vi "Send Command.vi"(8 "error in (no error)":errorcluster, 10 "write buffer":string, 11 "VISA resource name In":refnum<visa-resource-name>) -> (0 "error out":errorcluster, 3 "VISA resource name out":refnum<visa-resource-name>)   [LabVIEW 2017, in "Newport 1830-C.lvlib"]
doc: "Sends a command using the VISA drivers then waits sepecified ms."
uses:
  Newport 1830-C.lvlib
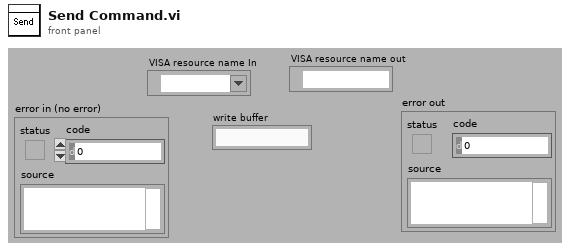
[diagram p1: front panel]
types:
  T1 = typedef "Semaphore RefNum" = refnum<k1>
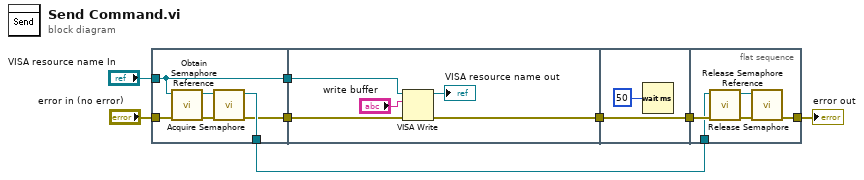
[diagram p0: block diagram]
diagram:
  n1 = flat-sequence {
    tunnel: "VISA resource name In" -> [w9]
    tunnel: [w9] -> w4
    tunnel: [w11] -> w3
    tunnel: [w12] -> w2
    tunnel: "error in (no error)" -> [w10]
    tunnel: [w15] -> w6
    tunnel: w4 -> [w17]
    tunnel: w3 -> [w16]
    tunnel: [w21] -> w7
    tunnel: w6 -> [w21]
    tunnel: w7 -> [w26]
    tunnel: w2 -> [w25]
    tunnel: [w22] -> w5
    frame #0 {
      n2 = call <vilib>:"Obtain Semaphore Reference.vi"("error in (no error)"=w10, "name (unnamed)"=w9) -> ("error out"=w13:errorcluster, "semaphore"=w14:T1)  [unwired: 3 in, 1 out]
      n3 = call <vilib>:"Acquire Semaphore.vi"("error in (no error)"=w13, "semaphore"=w14) -> ("error out"=w11:errorcluster, "semaphore out"=w12:T1)  [unwired: 3 in, 1 out]
    }
    frame #1 {
      n4 = VISA Write(VISA resource name=w17, write buffer="write buffer", error in (no error)=w16) -> (VISA resource name out=→"VISA resource name out":refnum<visa-resource-name>, error out=w15:errorcluster)  [unwired: 1 out]
    }
    frame #2 {
      n5 = Wait (ms)(milliseconds to wait=u32 50) -> ()  [unwired: 1 out]
    }
    frame #3 {
      n6 = call <vilib>:"Release Semaphore.vi"("error in (no error)"=w26, "semaphore"=w25) -> ("error out"=w24:errorcluster, "semaphore out"=w23:T1)  [unwired: 4 in]
      n7 = call <vilib>:"Release Semaphore Reference.vi"("error in (no error)"=w24, "semaphore"=w23) -> ("error out"=w22:errorcluster)  [unwired: 8 in, 1 out]
    }
  }
  "error out" <- w5
